vi "Set AI Settings by AI TaskName in Dict.vi"(8 "error in (no error)":errorcluster, 9 "AI Settings":T1, 10 "AI TaskName":string, 11 "DAQ":refnum<class "DAQ.lvclass">) -> (0 "error out":errorcluster, 1 "AI Settings out":T1, 3 "DAQ":refnum<class "DAQ.lvclass">)   [LabVIEW 2017, in "DAQ.lvclass"]
doc: "Developed by Kevin Thompson\nkevin@thompsonengineering.net\n\nCopyright 2018-2020\nThompson Engineering, LLC"
uses:
  DAQ.lvclass
  DataTypes/TD AI Instrument Settings--cluster.ctl
  DataTypes/TD AI InstSettings--cluster.ctl
  Process/ProcessSupport/TD SimAI Ranges--cluster.ctl
  DAQ.lvclass/DAQ.ctl
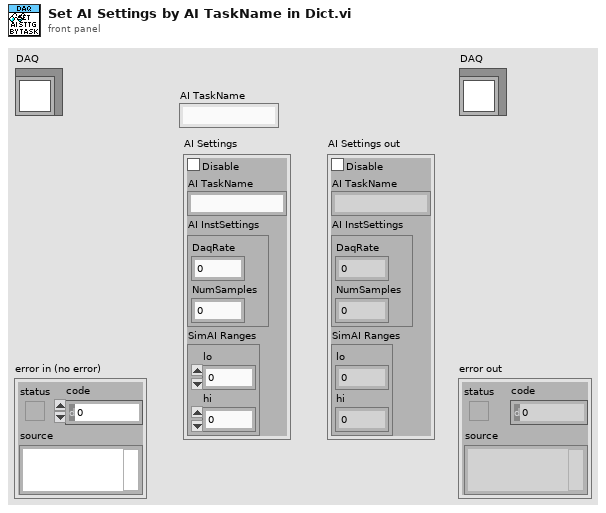
[diagram p1: front panel]
types:
  T1 = typedef "DAQ.lvclass/TD AI Instrument Settings--cluster.ctl" = cluster{"Disable":bool, "AI TaskName":string, "AI InstSettings":T2, "SimAI Ranges":T3}
  T2 = typedef "DAQ.lvclass/TD AI InstSettings--cluster.ctl" = cluster{"DaqRate":dbl, "NumSamples":i32}
  T3 = typedef "DAQ.lvclass/TD SimAI Ranges--cluster.ctl" = cluster{"lo":dbl, "hi":dbl}
  T4 = typedef "TD Dynamic CVT DVR--ref.ctl" = refnum<data-value>
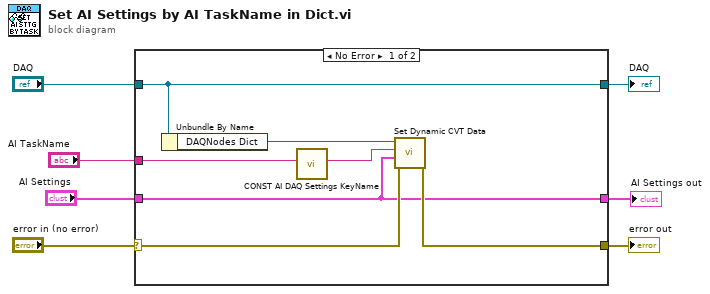
[diagram p0: block diagram]
diagram:
  n1 = case shown="No Error" "error in (no error)" {
    selector: "error in (no error)" -> [w11 w16]
    tunnel: [w9 w16] -> w6
    tunnel: [w14 w17] -> w4
    tunnel: "DAQ" -> [w14 w17]
    tunnel: "AI TaskName" -> [w13 _]
    tunnel: "AI Settings" -> [w8 w15]
    tunnel: [w8 w15] -> w1
    frame No Error {
      n2 = Unbundle By Name(w14) -> ("DAQNodes Dict"=w12:T4)
      n3 = call "CONST AI DAQ Settings KeyName.vi"("AI TaskName"=w13) -> ("AI DAQ Settings (KeyName)"=w10:string)  [unwired: 10 in]
      n4 = call <vilib>:"Set Dynamic CVT Data.vi"("error in (no error)"=w11, "value"=w8, "DataName"=w10, "dCVT DVR"=w12) -> ("error out"=w9:errorcluster)  [unwired: 5 in, 2 out]
    }
    frame Error {
    }
  }
  "error out" <- w6
  "DAQ" <- w4
  "AI Settings out" <- w1
